vi "PFI-28000-Chan-Bridge_Get Mute.vi"(8 "error in (no error)":errorcluster, 11 "PFI-28000-Chan-Bridge in":refnum<class "PFI-28000-Chan-Bridge.lvclass">) -> (0 "error out":errorcluster, 2 "Bypass":bool, 3 "PFI-28000-Chan-Bridge out":refnum<class "PFI-28000-Chan-Bridge.lvclass">)   [LabVIEW 2017, in "PFI-28000-Chan-Bridge.lvclass"]
uses:
  PFI-28000-Chan-Bridge.lvclass
  C:/wc/07143 Precision Filters 28000 Support/Driver/source/Channel/PFI-28000-Channel.lvclass
  Utilities/PFI-28000-Utils.lvlib
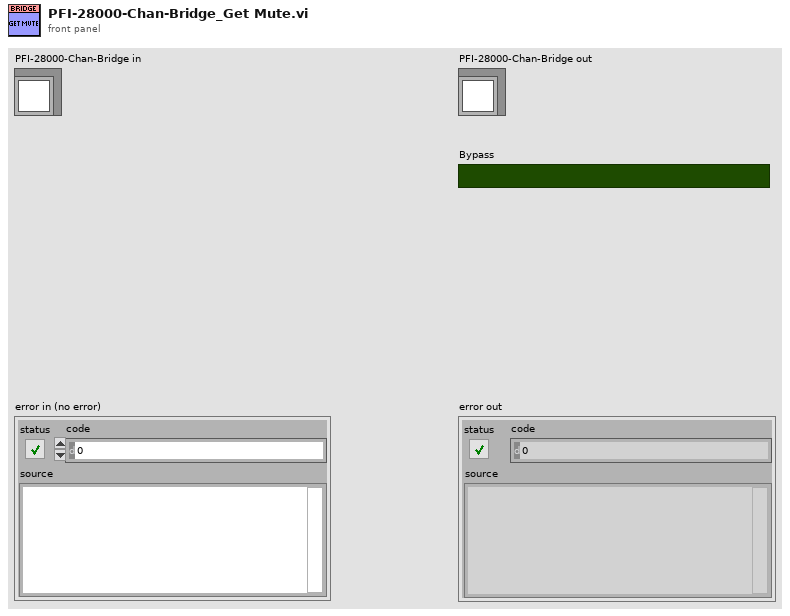
[diagram p1: front panel]
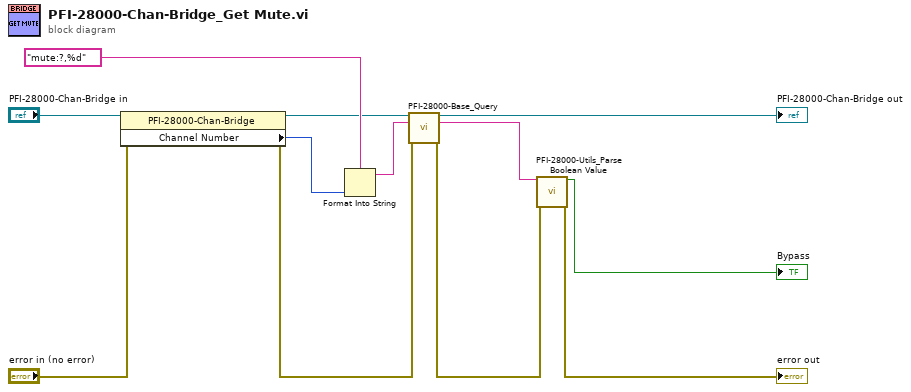
[diagram p0: block diagram]
diagram:
  n1 = property class="PFI-28000-Chan-Bridge"(reference="PFI-28000-Chan-Bridge in", error in="error in (no error)") -> (reference out=w6:refnum<class "PFI-28000-Chan-Bridge.lvclass">, error out=w3:errorcluster, "Channel Number"=w10:i32)
  n2 = Format Into String(format string="mute:?,%d" ("empty string"), w10) -> (resulting string=w4:string)  [unwired: 2 in, 1 out]
  n3 = call-dynamic "PFI-28000-Base_Query.vi"("PFI-28000-Base in"=w6, "Command"=w4, "error in (no error)"=w3) -> ("PFI-28000-Base out"=→"PFI-28000-Chan-Bridge out":refnum<class "PFI-28000-Chan-Bridge.lvclass">, "Response"=w2:string, "error out"=w1:errorcluster)  [unwired: 9 in, 1 out]
  n4 = call "PFI-28000-Utils_Parse Boolean Value.vi"("String"=w2, "error in (no error)"=w1) -> ("Value"=→"Bypass":bool, "error out"=→"error out":errorcluster)  [unwired: 12 in]
